vi "filter.vi"(10 "Temp":T1={"Vibr Chn Name"=[], "Analysis Chn Number"=0, "Index Vibration Waveform"={"t0"=timestamp(0 s since 1904-01-01), "dt"=1.0, "Y"=[]}, "Report Infomation"={"Test Name"="", "Tester"="", "Tempre Chart"=refnum, "Apli-Fre"=refnum, "Phase-Fre"=refnum, "Raw Data"=refnum}, "Vibr Apli - Fre"=[], "Vibr Phase - Fre"=[], "Error"={"status"=FALSE, "code"=0, "source"=""}, "Read Chan Name"="", "Test Info"={"Test Name"="", "Tester"=""}, "test data"=[{"t0"=timestamp(0 s since 1904-01-01), "dt"=1.0, "Y"=[]}, {"t0"=timestamp(0 s since 1904-01-01), "dt"=1.0, "Y"=[]}, {"t0"=timestamp(0 s since 1904-01-01), "dt"=1.0, "Y"=[]}, {"t0"=timestamp(0 s since 1904-01-01), "dt"=0.001, "Y"=[]}], "测试头文件"={"ch"=[], "测试环境"=""}, "CAl VAlUE"={"max_t"=[], "max_V"=[], "start_t"=[], "start_V"=[], "distance"=[], "unit"=""}}, 11 "averaging time":dbl=0.002) -> (2 "Temp out":T1={"Vibr Chn Name"=[], "Analysis Chn Number"=0, "Index Vibration Waveform"={"t0"=timestamp(0 s since 1904-01-01), "dt"=1.0, "Y"=[]}, "Report Infomation"={"Test Name"="", "Tester"="", "Tempre Chart"=refnum, "Apli-Fre"=refnum, "Phase-Fre"=refnum, "Raw Data"=refnum}, "Vibr Apli - Fre"=[], "Vibr Phase - Fre"=[], "Error"={"status"=FALSE, "code"=0, "source"=""}, "Read Chan Name"="", "Test Info"={"Test Name"="", "Tester"=""}, "test data"=[{"t0"=timestamp(0 s since 1904-01-01), "dt"=1.0, "Y"=[]}, {"t0"=timestamp(0 s since 1904-01-01), "dt"=1.0, "Y"=[]}, {"t0"=timestamp(0 s since 1904-01-01), "dt"=1.0, "Y"=[]}, {"t0"=timestamp(0 s since 1904-01-01), "dt"=0.001, "Y"=[]}], "测试头文件"={"ch"=[], "测试环境"=""}, "CAl VAlUE"={"max_t"=[], "max_V"=[], "start_t"=[], "start_V"=[], "distance"=[], "unit"=""}})   [LabVIEW 2011]
uses:
  Ctrls/ana data.ctl
  <vilib>/measure/madcrms.llb/Averaged DC-RMS for 1 Chan.vi
  <vilib>/measure/NI_MAPro.lvlib
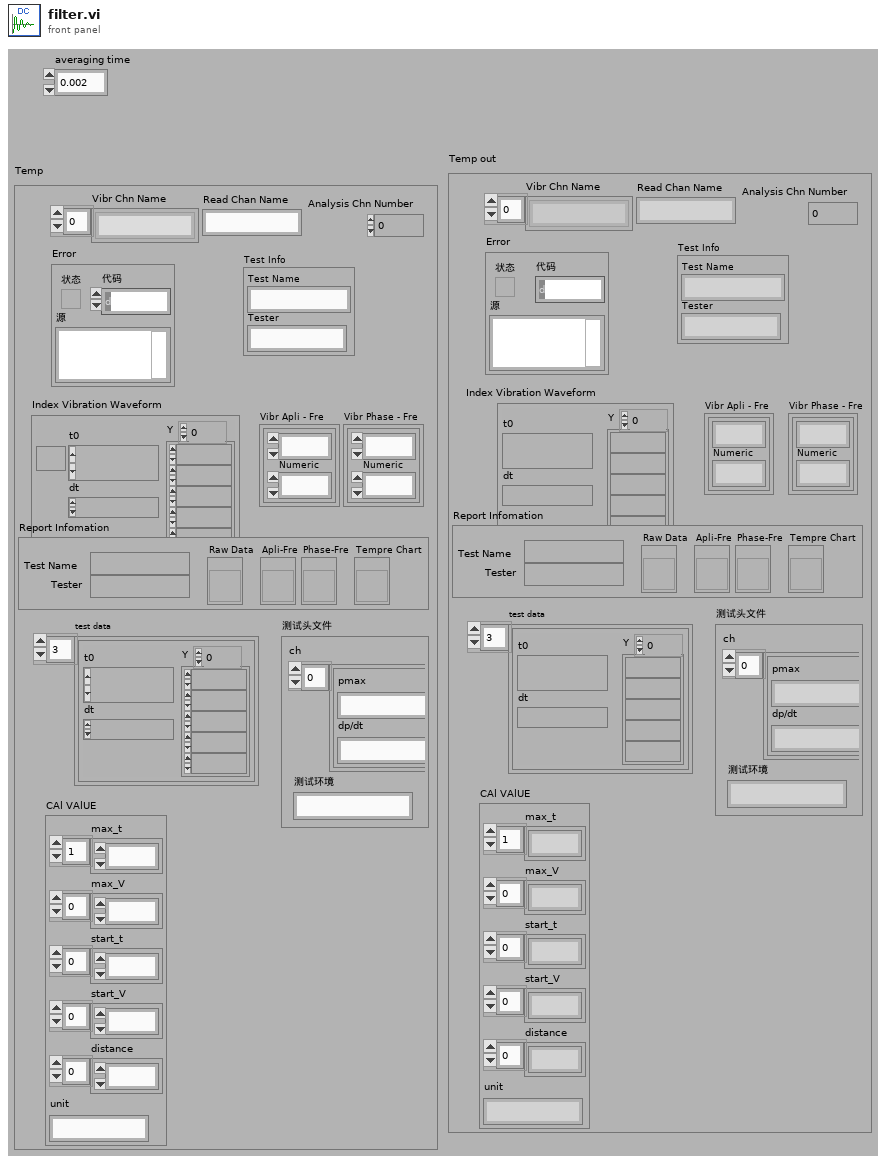
[diagram p1: front panel]
types:
  T1 = typedef "ana data.ctl" = cluster{"Vibr Chn Name":string[], "Analysis Chn Number":i32, "Index Vibration Waveform":waveform(dbl), "Report Infomation":cluster{"Test Name":string, "Tester":string, "Tempre Chart":refnum<vi>, "Apli-Fre":refnum<vi>, "Phase-Fre":refnum<vi>, "Raw Data":refnum<vi>}, "Vibr Apli - Fre":cluster{dbl, "Numeric":dbl}[], "Vibr Phase - Fre":cluster{dbl, "Numeric":dbl}[], "Error":errorcluster, "Read Chan Name":string, "Test Info":cluster{"Test Name":string, "Tester":string}, "test data":waveform(dbl)[], "测试头文件":cluster{"ch":cluster{"pmax":string, "dp/dt":string}[], "测试环境":string}, "CAl VAlUE":cluster{"max_t":dbl[], "max_V":dbl[], "start_t":dbl[], "start_V":dbl[], "distance":dbl[], "unit":string}}
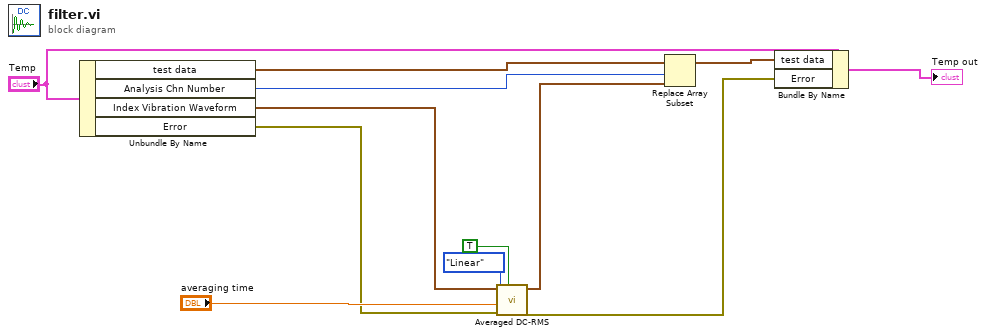
[diagram p0: block diagram]
diagram:
  n1 = Unbundle By Name("Temp") -> ("test data"=w9:waveform(dbl)[], "Analysis Chn Number"=w8:i32, "Index Vibration Waveform"=w10:waveform(dbl), "Error"=w3:errorcluster)
  n2 = call-poly <vilib>:"Averaged DC-RMS.vi"("reset"=TRUE, "error in (no error)"=w3, "averaging time"="averaging time", "averaging type"=enum16{"Linear", "Exponential"}."Linear", "signal in"=w10) -> ("error out"=w2:errorcluster, "DC value waveform"=w4:waveform(dbl))  [unwired: 1 in, 4 out]
  n3 = Replace Array Subset(array=w9, new element=w4, index=w8) -> (w5:waveform(dbl)[])
  n4 = Bundle By Name(cluster="Temp", "test data"=w5, "Error"=w2) -> (→"Temp out":T1)
